vi "Stopped.vi"(6 "Teller":refnum<class "Teller.lvclass">, 8 "Error in":errorcluster, 9 "Error":errorcluster, 10 "Unified Actor":refnum<class "Actor.lvclass">, 11 "Stopped jettl Msg in":refnum<class "Stopped jettl Msg.lvclass">) -> (0 "Error out":errorcluster, 3 "Stopped jettl Msg out":refnum<class "Stopped jettl Msg.lvclass">)   [LabVIEW 2020, in "jettl.lvlib" / "Stopped jettl Msg.lvlib" / "Stopped jettl Msg.lvclass"]
uses:
  Stopped jettl Msg.lvclass
  Actor/Actor.lvclass
  Teller/Teller.lvclass
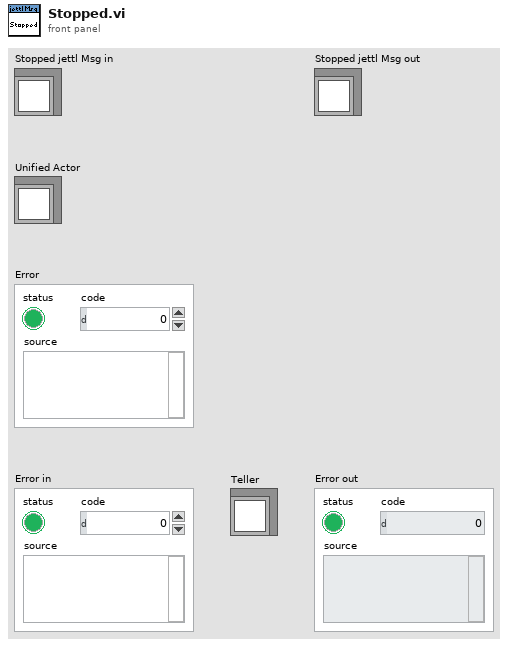
[diagram p1: front panel]
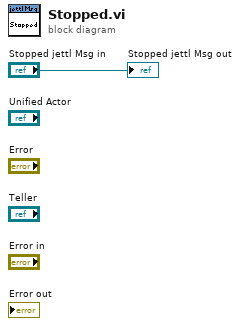
[diagram p0: block diagram]
diagram:
  "Stopped jettl Msg out" <- "Stopped jettl Msg in"
